vi "Windows Main-testComm.vi"() -> ()   [LabVIEW 2016]
panel:
  in  "testRadio":bool
  in  "testMode":bool
  in  "Stop":bool
  out "output array":u32[][](array[numeric])
  out "Image":T1(plugin-control)
  out "data out":u32[](array[numeric])
  in  "终端IP地址":string="192.168.48.235"
  out "error out":errorcluster
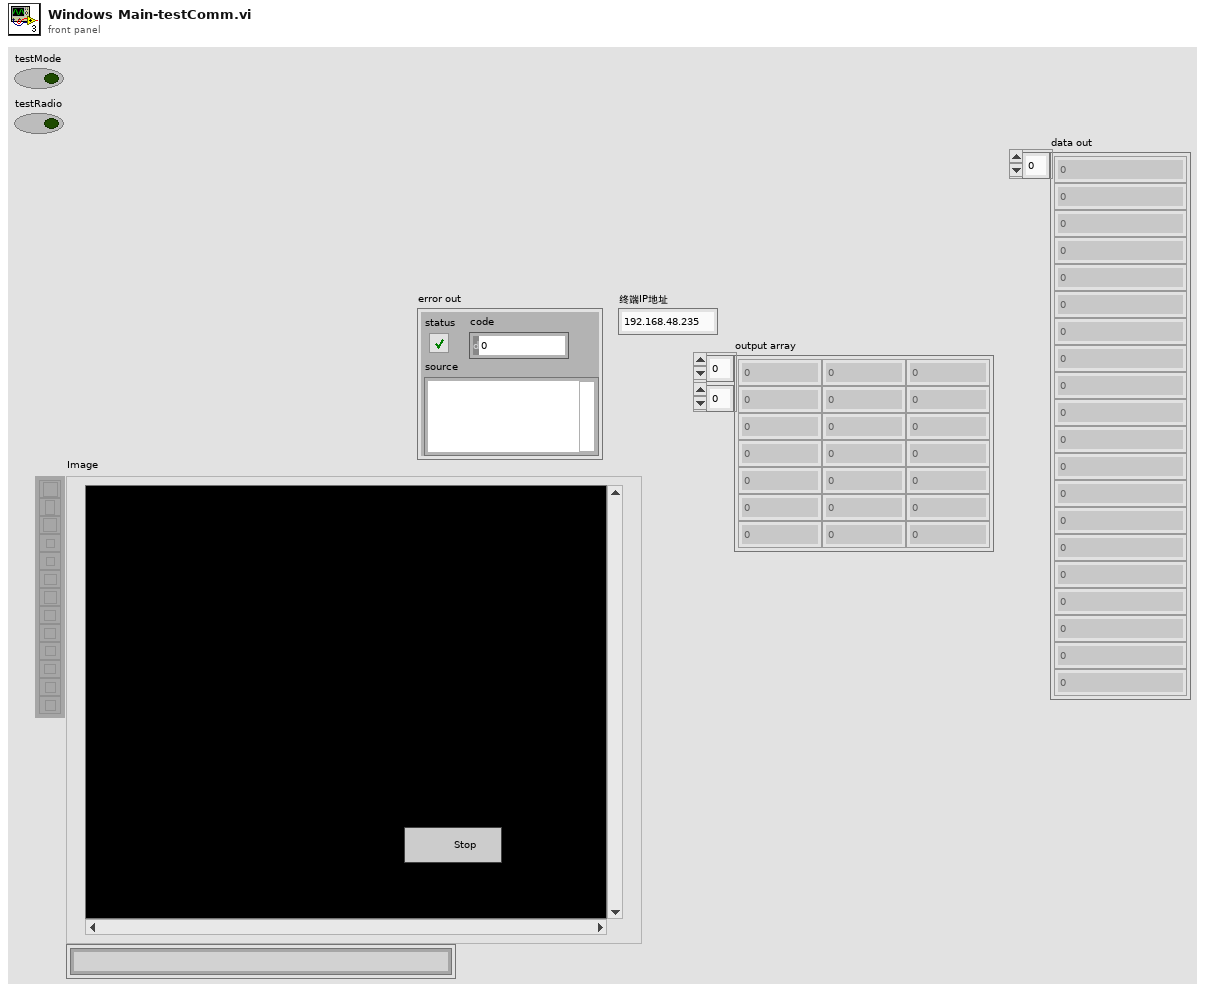
[diagram p1: front panel]
types:
  T1 = typedef "IMAQ Image.ctl" = refnum<image>
  T2 = typedef "Image Type" = u32
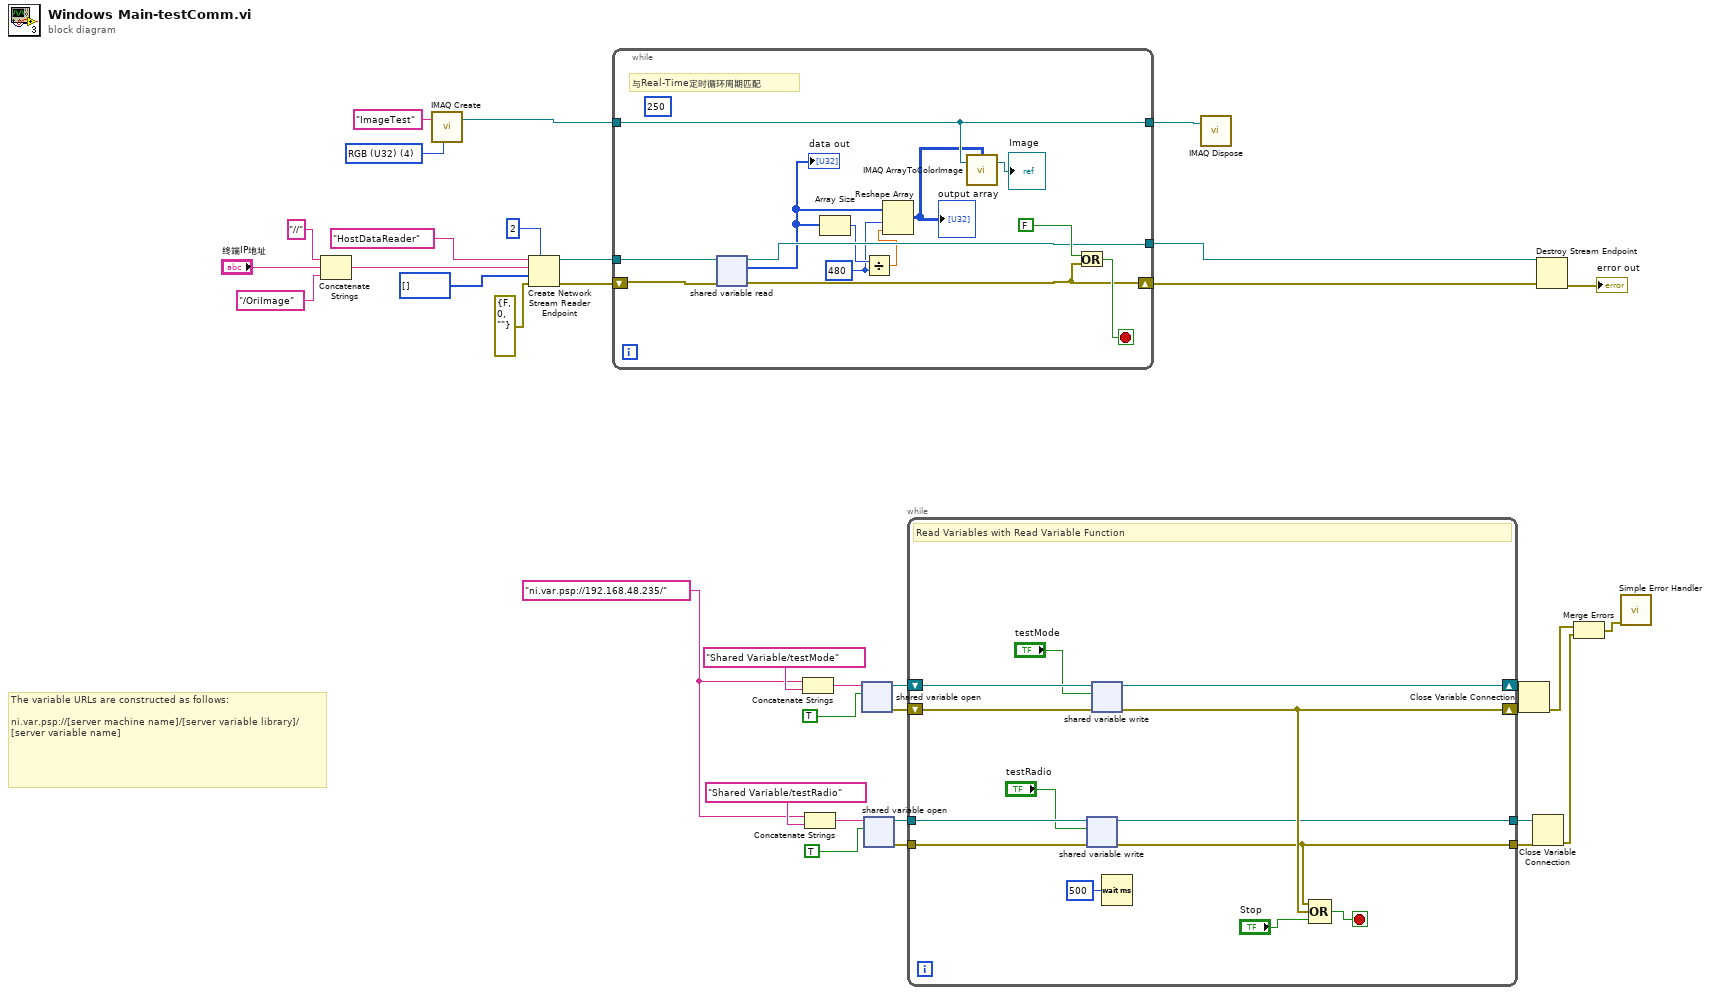
[diagram p0: block diagram]
diagram:
  w6 = "ni.var.psp://192.168.48.235/" ("string")
  w21 = T2 4 items=["Grayscale (U8)", "Grayscale (I16)", "Grayscale (SGL)", "Complex (CSG)", "RGB (U32)", "HSL (U32)", "RGB (U64)", "Grayscale (U16)"] ("Image Type")
  # "The variable URLs are constructed as follows:\n\nni.var.psp://[server machine name]/[server variable library]/[server variable name]"
  n1 = Concatenate Strings("//" ("string"), "终端IP地址", "/OriImage" ("string")) -> (w28:string)
  n2 = call "IMAQ Create"("Image Name"="ImageTest", "Image Type"=w21) -> ("New Image"=w20:T1)  [unwired: 3 in, 1 out]
  n3 = Create Network Stream Reader Endpoint(7:2 ("reader buffer size"), 8:errorcluster {"status"=FALSE, "code"=0, "source"=""} ("error in (no error)"), 9:i32[] [], 10:w28, 11:"HostDataReader" ("reader name")) -> (0:w35:errorcluster, 3:w26:refnum<k21>)  [unwired: 2 in]
  n4 = while {
    shift-right: [w45] -> w27
    shift-left: w35 -> [w46]
    tunnel: w26 -> [w44]
    tunnel: [w43] -> w25
    tunnel: w20 -> [w42]
    tunnel: [w42] -> w19
    stop <- w47 stop-if-true
    w40 = 480 ("y")
    (unwired) 250
    # "与Real-Time定时循环周期匹配"
    n5 = shared-variable-read(w44, w46) -> (w43:refnum<k21>, w45:errorcluster, w38:i32[])  [unwired: 1 in, 1 out]
    "data out" <- w38
    n6 = Array Size(array=w38) -> (size(s)=w41:i32)
    n7 = Divide(x=w41, y=w40) -> (x/y=w39:dbl)
    n8 = Reshape Array(w38, w40, w39) -> (w37:i32[][])
    "output array" <- w37
    n9 = call "IMAQ ArrayToColorImage"("Image Pixels (U32)"=w37, "Image"=w42) -> ("Image Out"=→"Image":T1)  [unwired: 3 in, 1 out]
    n10 = Or(x=FALSE ("停止应用程序"), y=w45) -> (x .or. y?=w47:bool)
  }
  n11 = Concatenate Strings(w6, "Shared Variable/testMode") -> (w15:string)
  n12 = Concatenate Strings(w6, "Shared Variable/testRadio") -> (w8:string)
  n13 = shared-variable-open(w15, TRUE) -> (w11:refnum<k21>, w12:errorcluster)  [unwired: 2 in]
  n14 = shared-variable-open(w8, TRUE) -> (w5:refnum<k21>, w4:errorcluster)  [unwired: 2 in]
  n15 = while {
    shift-right: [w57] -> w13
    shift-left: w11 -> [w58]
    shift-right: [w56] -> w14
    shift-left: w12 -> [w59]
    tunnel: w5 -> [w54]
    tunnel: w4 -> [w53]
    tunnel: [w51] -> w3
    tunnel: [w50] -> w2
    stop <- w60 stop-if-true
    # "Read Variables with Read Variable Function"
    n16 = shared-variable-write(w54, w53, "testRadio") -> (w51:refnum<k21>, w50:errorcluster)
    n17 = shared-variable-write(w58, w59, "testMode") -> (w57:refnum<k21>, w56:errorcluster)
    n18 = Wait (ms)(milliseconds to wait=u32 500 ("millisecond multiple")) -> ()  [unwired: 1 out]
    n19 = Compound Arithmetic op=OR(w50, w56, "Stop") -> (w60:bool)
  }
  n20 = call "IMAQ Dispose"("Image"=w19) -> ()  [unwired: 5 in, 1 out]
  n21 = Close Variable Connection(8:w14, 11:w13) -> (0:w18:errorcluster)
  n22 = Close Variable Connection(8:w2, 11:w3) -> (0:w1:errorcluster)
  n23 = Destroy Stream Endpoint(8:w27, 11:w25) -> (0:→"error out":errorcluster)
  n24 = Merge Errors(w18, w1) -> (w17:errorcluster)
  n25 = call <vilib>:"Simple Error Handler.vi"("error in (no error)"=w17) -> ()  [unwired: 4 in, 5 out]
